vi "GetControlValue [Poly].vi"   [LabVIEW 2016, in "Drona.lvlib" / "GetControlValue.lvlib"]
uses:
  GetControlValue/GetControlValue.lvlib
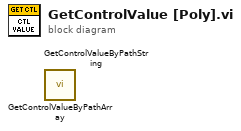
[diagram p0: block diagram]
diagram:
  n1 = call "GetControlValueByPathArray.vi"() -> ()  [unwired: 13 in, 3 out]
  n2 = call "GetControlValueByPathString.vi"() -> ()  [unwired: 13 in, 3 out]
